vi "Apply special move.vi"(8 "error in (no error)":errorcluster, 10 "Position in":refnum<class "Position.lvclass">, 11 "Move in":refnum<class "Move.lvclass">) -> (0 "error out":errorcluster, 2 "Position out":refnum<class "Position.lvclass">, 3 "Move out":refnum<class "Move.lvclass">)   [LabVIEW 2015, in "Chesslib.lvlib" / "Move.lvclass"]
uses:
  Move.lvclass
  Position/Position.lvclass
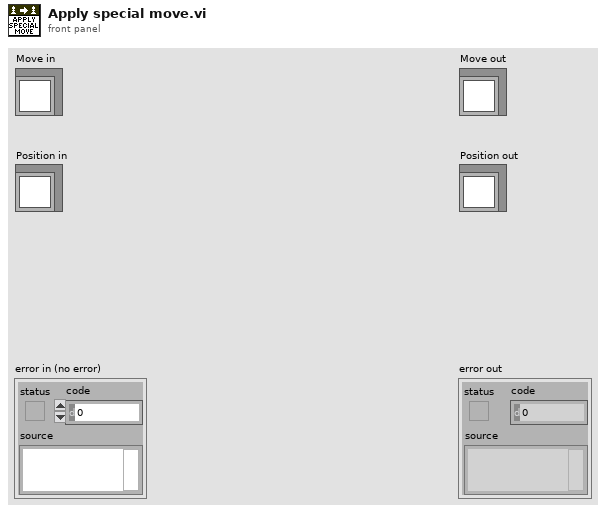
[diagram p1: front panel]
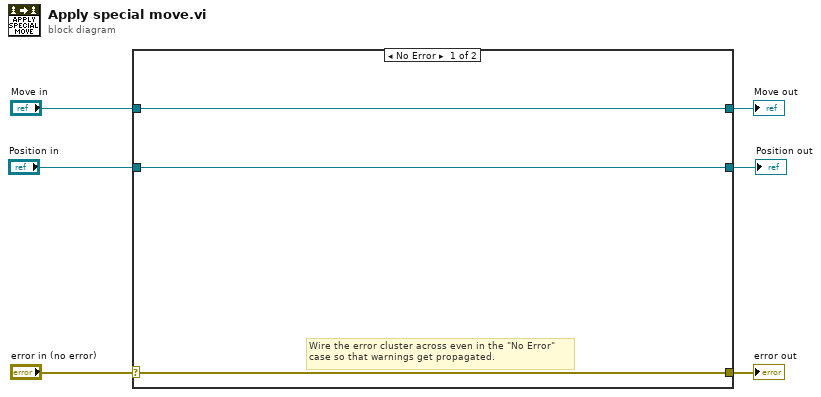
[diagram p0: block diagram]
diagram:
  n1 = case shown="No Error" "error in (no error)" {
    selector: "error in (no error)" -> [w8 w12]
    tunnel: [w8 w12] -> w5
    tunnel: [w9 w11] -> w3
    tunnel: "Move in" -> [w9 w11]
    tunnel: "Position in" -> [w7 w10]
    tunnel: [w7 w10] -> w1
    frame No Error {
      # "Wire the error cluster across even in the \"No Error\"\ncase so that warnings get propagated."
    }
    frame Error {
    }
  }
  "error out" <- w5
  "Move out" <- w3
  "Position out" <- w1
